vi "tm452_recordanddisplay_wVision.vi"() -> ()   [LabVIEW 2011]
panel:
  out "Frames Recorded":i32
  in  "Frames":i32=100
  in  "DCIMG Path":path
  out "Display":T1(plugin-control)
  out "DCAM Version":string
  out "Library Version":string
  out "Error Out":errorcluster {"code" format="%.0x"}
  # "This is an example of how to use the\nhard disk recorder functions to record\nimages to a DCIMG file and display\nimages as you are recording."
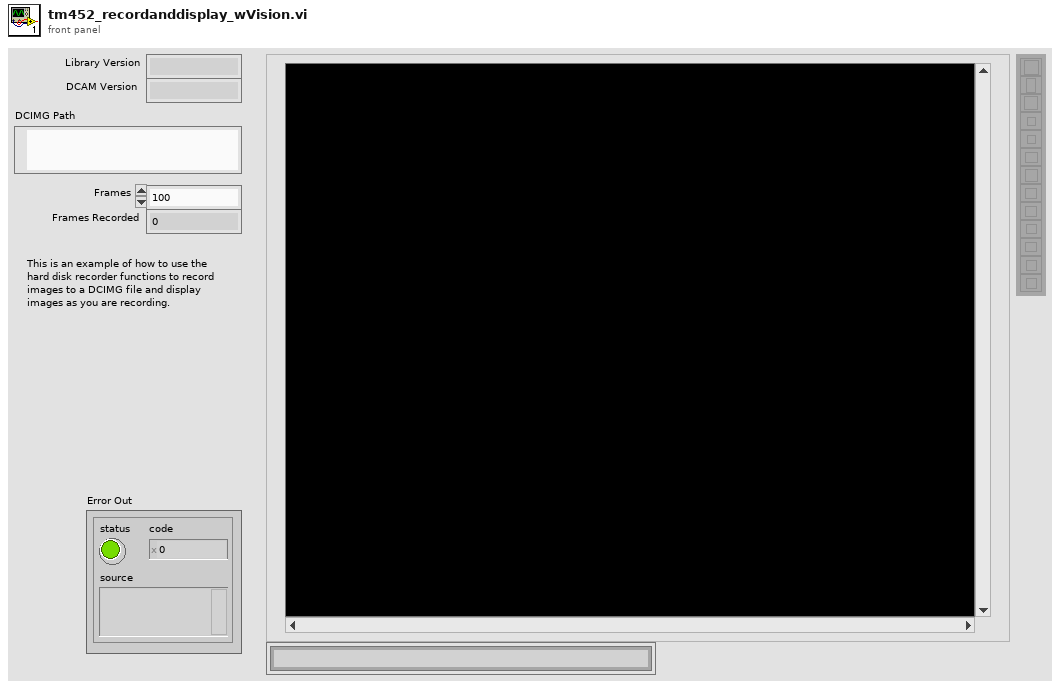
[diagram p1: front panel]
types:
  T1 = typedef "IMAQ Image.ctl" = refnum<image>
  T2 = cluster{"Capture Library":string, "DCAM-API":string}
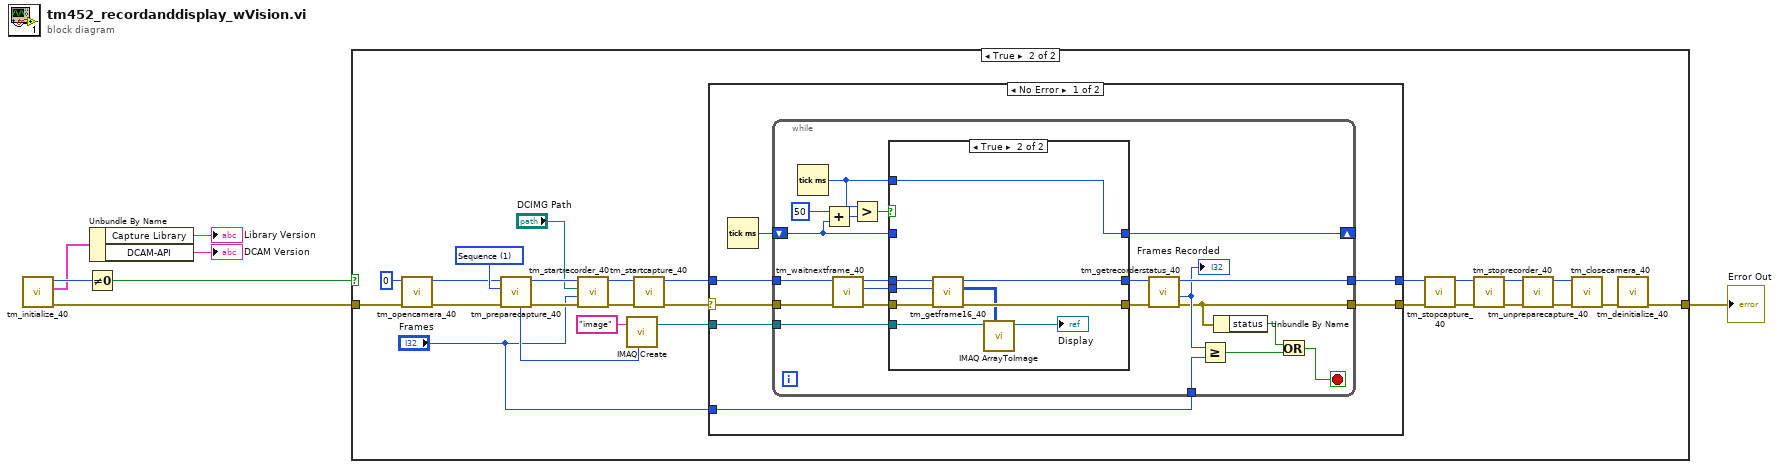
[diagram p0: block diagram]
diagram:
  n1 = call <userlib>:"tm_initialize_40.vi"() -> ("error out"=w4:errorcluster, "Version Info"=w3:T2, "Number Of Cameras"=w5:u32)  [unwired: 8 in, 1 out]
  n2 = Not Equal To 0?(x=w5) -> (x != 0?=w7:bool)
  n3 = Unbundle By Name(w3) -> ("Capture Library"=→"Library Version":string, "DCAM-API"=→"DCAM Version":string)
  n4 = case shown="True" w7 {
    tunnel: w4 -> [w8 w34]
    tunnel: [w8 w31] -> w6
    frame False {
    }
    frame True {
      w28 = 1 items=["Snap", "Sequence"] ("Capture mode")
      n5 = call <userlib>:"tm_opencamera_40.vi"("error in (no error)"=w34, "Camera Index"=u32 0) -> ("error out"=w26:errorcluster, "Handle out"=w27:u32)  [unwired: 7 in, 1 out]
      n6 = call <userlib>:"tm_preparecapture_40.vi"("error in (no error)"=w26, "Capture mode"=w28, "Handle in"=w27) -> ("error out"=w23:errorcluster, "Handle out"=w24:u32, "Image type"=w12:u32)  [unwired: 5 in, 1 out]
      n7 = call <userlib>:"tm_startrecorder_40.vi"("error in (no error)"=w23, "frames"="Frames", "File"="DCIMG Path", "Handle in"=w24) -> ("error out"=w22:errorcluster, "Handle out"=w21:u32)  [unwired: 6 in]
      n8 = call "IMAQ Create"("Image Name"="image", "Image Type"=w12) -> ("New Image"=w13:T1)  [unwired: 3 in, 1 out]
      n9 = call <userlib>:"tm_startcapture_40.vi"("error in (no error)"=w22, "Handle in"=w21) -> ("error out"=w15:errorcluster, "Handle out"=w14:u32)  [unwired: 8 in]
      n10 = case shown="No Error" w15 {
        selector: w15 -> [w40 w75]
        tunnel: w14 -> [w39 w76]
        tunnel: w13 -> [w38 _]
        tunnel: "Frames" -> [w37 _]
        tunnel: [w36 w76] -> w10
        tunnel: [w35 w75] -> w9
        frame No Error {
          n11 = Tick Count (ms)() -> (millisecond timer value=w41:u32)
          n12 = while {
            tunnel: [w48] -> w36
            tunnel: [w45] -> w35
            tunnel: w39 -> [w61]
            tunnel: w40 -> [w62]
            shift-right: [w52] -> _
            shift-left: w41 -> [w53]
            tunnel: w38 -> [w51]
            tunnel: w37 -> [w46]
            stop <- w42 stop-if-true
            n13 = Tick Count (ms)() -> (millisecond timer value=w54:u32)
            n14 = Add(x=u32 50, y=w53) -> (x+y=w56:u32)
            n15 = call <userlib>:"tm_waitnextframe_40.vi"("error in (no error)"=w62, "Handle in"=w61) -> ("error out"=w59:errorcluster, "Frame Index"=w58:i32, "Handle out"=w60:u32)  [unwired: 6 in, 1 out]
            n16 = Greater?(x=w54, y=w56) -> (0:w55:bool)
            n17 = case shown="True" w55 {
              tunnel: w60 -> [w65 w74]
              tunnel: w59 -> [w64 w73]
              tunnel: w58 -> [_ w66]
              tunnel: w53 -> [w63 _]
              tunnel: w54 -> [_ w72]
              tunnel: [w65 w70] -> w50
              tunnel: [w64 w71] -> w49
              tunnel: [w63 w72] -> w52
              tunnel: w51 -> [_ w68]
              frame False {
              }
              frame True {
                n18 = call <userlib>:"tm_getframe16_40.vi"("error in (no error)"=w73, "Frame Index"=w66, "Handle in"=w74) -> ("error out"=w71:errorcluster, "Data"=w69:u16[][], "Handle out"=w70:u32)  [unwired: 5 in, 1 out]
                n19 = call "IMAQ ArrayToImage"("Image Pixels (U16)"=w69, "Image"=w68) -> ("Image Out"=→"Display":T1)  [unwired: 8 in, 1 out]
              }
            }
            n20 = call <userlib>:"tm_getrecorderstatus_40.vi"("error in (no error)"=w49, "Handle"=w50) -> ("error out"=w45:errorcluster, "Count"=w47:i32, "Handle"=w48:u32)  [unwired: 6 in, 1 out]
            "Frames Recorded" <- w47
            n21 = Greater Or Equal?(x=w47, y=w46) -> (x >= y?=w43:bool)
            n22 = Unbundle By Name(w45) -> ("status"=w44:bool)
            n23 = Or(x=w44, y=w43) -> (x .or. y?=w42:bool)
          }
        }
        frame Error {
        }
      }
      n24 = call <userlib>:"tm_stopcapture_40.vi"("error in (no error)"=w9, "Handle in"=w10) -> ("error out"=w19:errorcluster, "Handle out"=w18:u32)  [unwired: 8 in]
      n25 = call <userlib>:"tm_stoprecorder_40.vi"("error in (no error)"=w19, "Handle in"=w18) -> ("error out"=w16:errorcluster, "Handle out"=w17:u32)  [unwired: 8 in]
      n26 = call <userlib>:"tm_unpreparecapture_40.vi"("error in (no error)"=w16, "Handle in"=w17) -> ("error out"=w30:errorcluster, "Handle out"=w29:u32)  [unwired: 8 in]
      n27 = call <userlib>:"tm_closecamera_40.vi"("error in (no error)"=w30, "Handle in"=w29) -> ("error out"=w32:errorcluster)  [unwired: 9 in]
      n28 = call <userlib>:"tm_deinitialize_40.vi"("error in (no error)"=w32) -> ("error out"=w31:errorcluster)  [unwired: 10 in]
    }
  }
  "Error Out" <- w6
